vi "Detect feature translation between images.vi"(0 "Test image file path":path=path "C:/Users/Paul Nathan/Desktop/Building test pictures/Building_pos_1.jpg", 1 "ROI to crop (pixels)":T2={"Xmax"=2147483647, "Ymax"=2147483647, "Xmin"=0, "Ymin"=0}, 2 "Txy range (pixels)":T1={"Tx max (pix)"=2147483647, "Tx min (pix)"=-2147483648, "Ty max (pix)"=2147483647, "Ty min (pix)"=-2147483648}, 3 "Max iters":i32=10000, 4 "Grad step (pix)":dbl=0.01 format="%#_13g", 5 "tol^2 (pix^2)":dbl=1e-09 format="%#_13g", 6 "Reference image file path":path=path "C:/Users/Paul Nathan/Desktop/Building test pictures/Building_pos_1.jpg", 7 "Error In":errorcluster) -> (13 "Error out":errorcluster, 14 "dx (pix)":dbl, 15 "dy (pix)":dbl, 18 "Sub-pixel convergence":bool, 19 "Iterations":i32)   [LabVIEW 2015]
uses:
  Typedefs/ROI bounds.ctl
  Typedefs/Txy range.ctl
  <vilib>/Analysis/2dsp.llb/2D Cross Correlation (CDB).vi
  <vilib>/Analysis/baseanly.llb/Scale 2D.vi
  <vilib>/Analysis/NI_AALPro.lvlib
  <vilib>/Analysis/NI_AALBase.lvlib
panel:
  out "Xcorr function":dbl[][](graph)
  # "Paul Nathan 09/06/2015,\n21/03/2016"
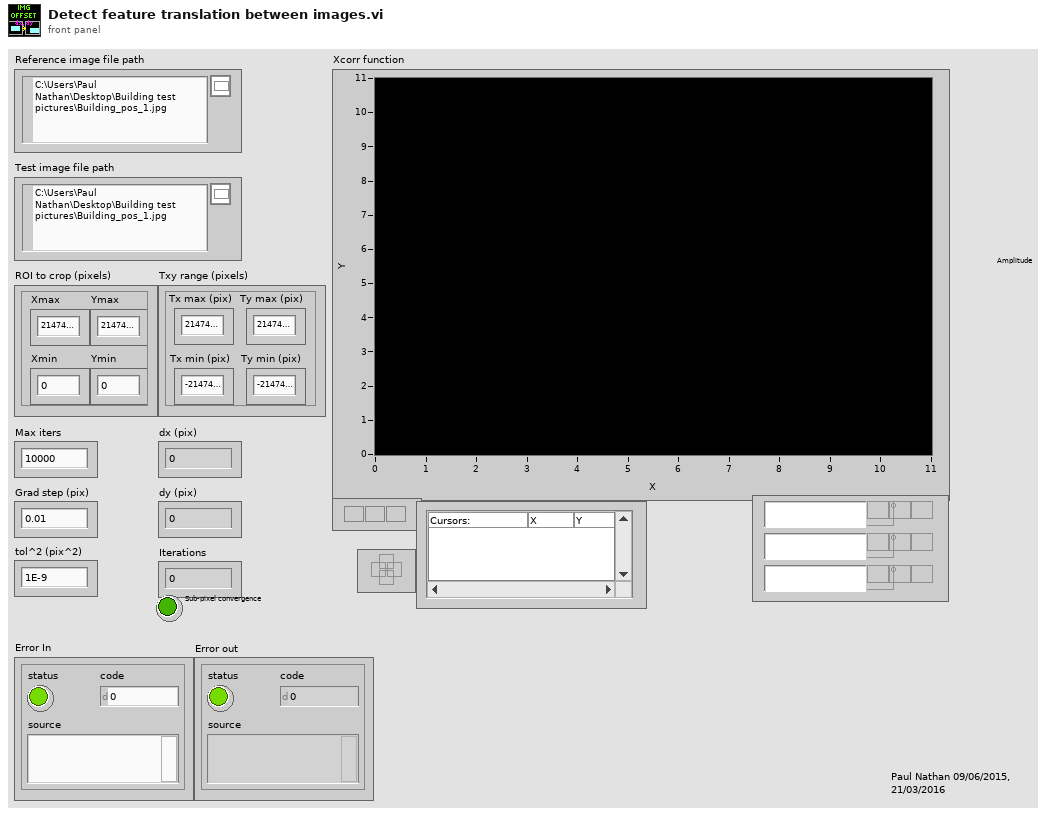
[diagram p1: front panel]
types:
  T1 = typedef "Txy range.ctl" = cluster{"Tx max (pix)":i32, "Tx min (pix)":i32, "Ty max (pix)":i32, "Ty min (pix)":i32}
  T2 = typedef "ROI bounds.ctl" = cluster{"Xmax":i32, "Ymax":i32, "Xmin":i32, "Ymin":i32}
  T3 = typedef "Image Type" = u32
  T4 = typedef "IMAQ Image.ctl" = refnum<image>
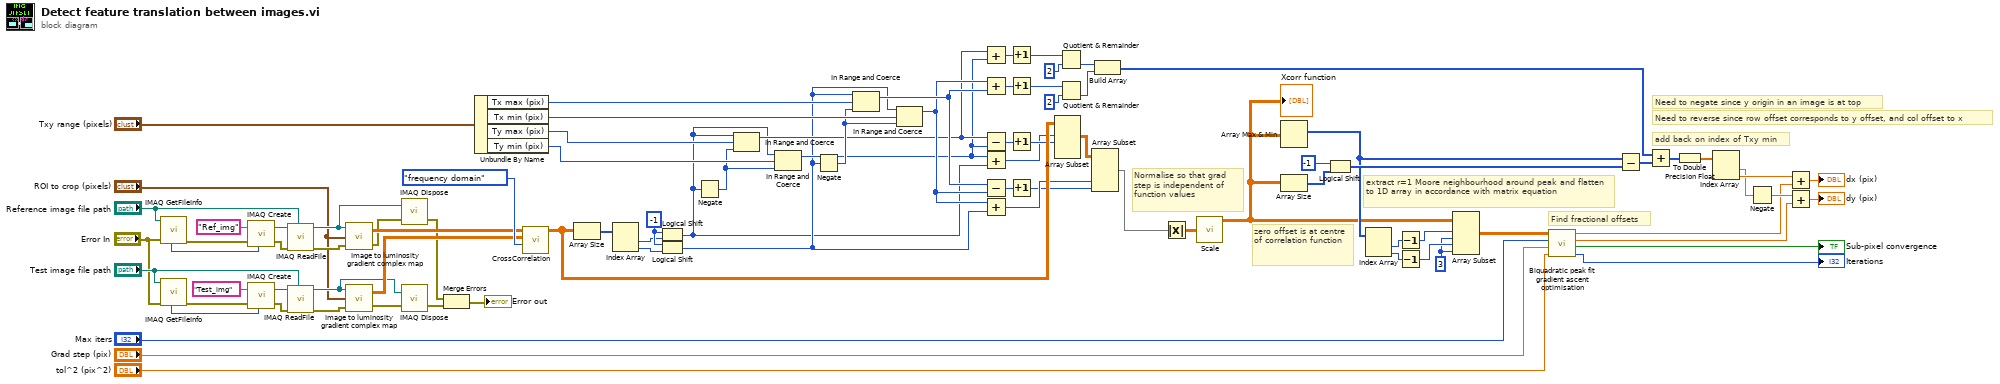
[diagram p0: block diagram]
diagram:
  w27 = i16 -1 ("y")
  w69 = 3 ("length")
  # "add back on index of Txy min"
  # "Normalise so that grad step is independent of function values"
  # "zero offset is at centre of correlation function"
  # "Need to reverse since row offset corresponds to y offset, and col offset to x"
  # "Need to negate since y origin in an image is at top"
  # "extract r=1 Moore neighbourhood around peak and flatten to 1D array in accordance with matrix equation"
  # "Find fractional offsets"
  n1 = call "IMAQ GetFileInfo"("error in (no error)"="Error In", "File Path"="Reference image file path") -> ("error out"=w85:errorcluster, "Image Type"=w79:T3)  [unwired: 3 in, 5 out]
  n2 = call "IMAQ GetFileInfo"("error in (no error)"="Error In", "File Path"="Test image file path") -> ("error out"=w83:errorcluster, "Image Type"=w84:T3)  [unwired: 3 in, 5 out]
  n3 = call "IMAQ Create"("Image Name"="Ref_img", "Image Type"=w79, "error in (no error)"=w85) -> ("New Image"=w87:T4, "error out"=w86:errorcluster)  [unwired: 2 in]
  n4 = call "IMAQ Create"("Image Name"="Test_img", "Image Type"=w84, "error in (no error)"=w83) -> ("New Image"=w81:T4, "error out"=w82:errorcluster)  [unwired: 2 in]
  n5 = call "IMAQ ReadFile"("File Path"="Reference image file path", "error in (no error)"=w86, "Image"=w87) -> ("error out"=w62:errorcluster, "Image Out"=w55:T4)  [unwired: 4 in, 3 out]
  n6 = call "IMAQ ReadFile"("File Path"="Test image file path", "error in (no error)"=w82, "Image"=w81) -> ("error out"=w61:errorcluster, "Image Out"=w57:T4)  [unwired: 4 in, 3 out]
  n7 = call "Image to luminosity gradient complex map.vi"("Error In"=w62, "ROI to crop (pixels)"="ROI to crop (pixels)", "Image"=w55) -> ("Error Out"=w56:errorcluster, "Luminosity gradient map (complex)"=w59:cdb[][])
  n8 = call "Image to luminosity gradient complex map.vi"("Error In"=w61, "ROI to crop (pixels)"="ROI to crop (pixels)", "Image"=w57) -> ("Error Out"=w58:errorcluster, "Luminosity gradient map (complex)"=w60:cdb[][])
  n9 = call "IMAQ Dispose"("Image"=w55, "error in (no error)"=w56) -> ("error out"=w53:errorcluster)  [unwired: 4 in]
  n10 = call "IMAQ Dispose"("Image"=w57, "error in (no error)"=w58) -> ("error out"=w54:errorcluster)  [unwired: 4 in]
  n11 = Merge Errors(w53, w54) -> (→"Error out":errorcluster)
  n12 = Unbundle By Name("Txy range (pixels)") -> ("Tx max (pix)"=w12:i32, "Tx min (pix)"=w11:i32, "Ty max (pix)"=w20:i32, "Ty min (pix)"=w25:i32)
  n13 = call-poly <vilib>:"CrossCorrelation.vi"("algorithm"=enum32{"direct", "frequency domain"}."frequency domain", "Y"=w60, "X"=w59) -> ("Rxy"=w33:cdb[][])  [unwired: 7 in, 1 out]
  n14 = Array Size(array=w33) -> (size(s)=w35:i32[])
  n15 = Index Array(array=w35) -> (element #1=w3:i32, element #2=w8:i32)  [unwired: 2 in]
  n16 = Logical Shift(y=w27, x=w3) -> (x << y=w1:i32)
  n17 = Logical Shift(y=w27, x=w8) -> (x << y=w2:i32)
  n18 = Negate(x=w1) -> (-x=w4:i32)
  n19 = In Range and Coerce(upper limit=w1, x=w20, lower limit=w4) -> (coerced(x)=w6:i32)  [unwired: 1 out]
  n20 = In Range and Coerce(upper limit=w1, x=w25, lower limit=w4) -> (coerced(x)=w5:i32)  [unwired: 1 out]
  n21 = Negate(x=w2) -> (-x=w7:i32)
  n22 = In Range and Coerce(upper limit=w2, x=w12, lower limit=w7) -> (coerced(x)=w10:i32)  [unwired: 1 out]
  n23 = In Range and Coerce(upper limit=w2, x=w11, lower limit=w7) -> (coerced(x)=w9:i32)  [unwired: 1 out]
  n24 = Add(x=w6, y=w5) -> (x+y=w24:i32)
  n25 = Add(x=w9, y=w10) -> (x+y=w14:i32)
  n26 = Subtract(x=w6, y=w5) -> (x-y=w36:i32)
  n27 = Add(x=w5, y=w1) -> (x+y=w26:i32)
  n28 = Subtract(x=w10, y=w9) -> (x-y=w19:i32)
  n29 = Add(x=w9, y=w2) -> (x+y=w29:i32)
  n30 = Increment(x=w24) -> (x+1=w21:i32)
  n31 = Increment(x=w14) -> (x+1=w16:i32)
  n32 = Increment(x=w36) -> (x+1=w31:i32)
  n33 = Increment(x=w19) -> (x+1=w18:i32)
  n34 = Array Subset(array=w33, index (row)=w26, length (row)=w31) -> (w34:cdb[][])  [unwired: 2 in]
  n35 = Quotient & Remainder(x=w21, y=2) -> (floor(x/y)=w22:i32)  [unwired: 1 out]
  n36 = Quotient & Remainder(x=w16, y=2) -> (floor(x/y)=w13:i32)  [unwired: 1 out]
  n37 = Array Subset(array=w34, index (col)=w29, length (col)=w18) -> (w32:cdb[][])  [unwired: 2 in]
  n38 = Build Array(w22, w13) -> (w17:i32[])
  n39 = Absolute Value(x=w32) -> (abs(x)=w64:dbl[][])
  n40 = call-poly <vilib>:"Scale.vi"("X"=w64) -> ("Y=(X-offset)/scale"=w63:dbl[][])  [unwired: 3 out]
  "Xcorr function" <- w63
  n41 = Array Max & Min(array=w63) -> (max index (indices)=w66:i32[])  [unwired: 3 out]
  n42 = Array Size(array=w63) -> (size(s)=w74:i32[])
  n43 = Logical Shift(y=i16 -1, x=w74) -> (x << y=w68:i32[])
  n44 = Index Array(array=w66) -> (element #1=w73:i32, element #2=w72:i32)  [unwired: 2 in]
  n45 = Decrement(x=w73) -> (x-1=w71:i32)
  n46 = Decrement(x=w72) -> (x-1=w70:i32)
  n47 = Array Subset(array=w63, index (row)=w71, length (row)=w69, index (col)=w70, length (col)=w69) -> (w47:dbl[][])
  n48 = call "Biquadratic peak fit gradient ascent optimisation.vi"("tol^2"="tol^2 (pix^2)", "Grad step"="Grad step (pix)", "Max iters"="Max iters", "3x3 peak patch"=w47) -> ("Iterations"=→"Iterations":i32, "Sub-pixel convergence"=→"Sub-pixel convergence":bool, "dy"=w42:dbl, "dx"=w43:dbl)
  n49 = Subtract(x=w66, y=w68) -> (x-y=w30:i32[])
  n50 = Add(x=w17, y=w30) -> (x+y=w28:i32[])
  n51 = To Double Precision Float(number=w28) -> (double precision float=w67:dbl[])
  n52 = Index Array(array=w67) -> (element #1=w49:dbl, element #2=w50:dbl)  [unwired: 2 in]
  n53 = Negate(x=w49) -> (-x=w48:dbl)
  n54 = Add(x=w50, y=w43) -> (x+y=→"dx (pix)":dbl)
  n55 = Add(x=w48, y=w42) -> (x+y=→"dy (pix)":dbl)
